vi "Fit Tilted Logistic Square Pulse.vi"(0 "Decay":T14, 5 "Boundaries":dbl[](array[numeric]), 9 "Basic Fit Options":T4, 11 "error in (no error)":errorcluster, 12 "Square Pulse Options":T2={"Method"=enum."Mode", "# Bins"=0, "Threshold %"=10.0, "Center on Midpoint"=TRUE, "Smoothen Plot"=FALSE}) -> (4 "Fitted Decay":cluster{"t Array":dbl[], "Fitted Array":dbl[]}, 6 "Residuals":cluster{"t Array":dbl[], "Residual Array":dbl[]}, 8 "Fit Output":T9={"best nonlinear fit"=[], "best fit parameters"=[], "R^2"=0.0, "RMSE"=0.0, "error out"={"status"=FALSE, "code"=0, "source"=""}, "Fitting Method"=enum."Least Square", "number of function calls"=0, "number of iterations"=0, "covariance"=[], "Chi 2"=0.0, "DOF"=0, "Fit Convergence Criterion"=enum."Continue", "Fitting Algorithm"=enum."Levenberg-Marquardt", "Weighted Fit"=enum."Unweighted", "Gradient"=0.0, "|Delta Chi 2|"=0.0, "|Delta Chi 2|/Chi 2"=0.0, "Max |Delta a| /|a|"=0.0, "Lambda"=-1.0, "RSS"=0.0, "AIC"=0.0, "BIC"=0.0, "Max number of function calls"=0, "Max number of iterations"=0, "IRF"={"X Array"=[], "Y Array"=[]}, "IRF Normalization Factor"=0.0, "Decay Normalization Factor"=0.0, "Number of offset fits"=0, "Weighted Chi2"=-1.0, "Unweighted Chi2"=-1.0}, 10 "Delta Best Fit Parameters":dbl[](array[numeric]), 15 "error out":errorcluster)   [LabVIEW 2021, in "Fits.lvlib"]
uses:
  Fits.lvlib
  Time/Time.lvlib
  <vilib>/ErrorRing/Error Ring.xnode
  <vilib>/Utility/error.llb/DialogType.ctl
  LM model Function and gradient (Tilted Logistic Square-Gated IRF).vi
  <vilib>/Utility/error.llb/Error Cluster From Error Code.vi
  Arrays/Arrays.lvlib
  Graphs/XY Graph/XY Graph Plot Data.ctl
  Graphs/XY Graph/XY Graph Add-Ons.lvlib
  Decay Convolution/Fit Control Data.ctl
  <vilib>/Analysis/Matrix/Datatypes/RealMatrix.ctl
  <vilib>/Analysis/Matrix/NI_Matrix.lvlib
  Non-linear Fit Output v4.ctl
  Residual Type.ctl
  Basic Fit Options.ctl
  Square Pulse Levels Type.ctl
  Square Pulse Options.ctl
  Convergence Criteria.ctl
  Non-linear Fitting Algorithm.ctl
  Non-linear Fitting Method v2.ctl
  Nonlinear Fit Method.ctl
  Optimal Offset Selection Criterion.ctl
  IRF(X)PSED/Fit Weights Type v2.ctl
panel:
  in  "Optimal Offset Selection Criterion":T1
  out "XY Graph":cluster{"X Array":dbl[], "Y Array":dbl[]}[](graph)
  out "CPU (s)":dbl
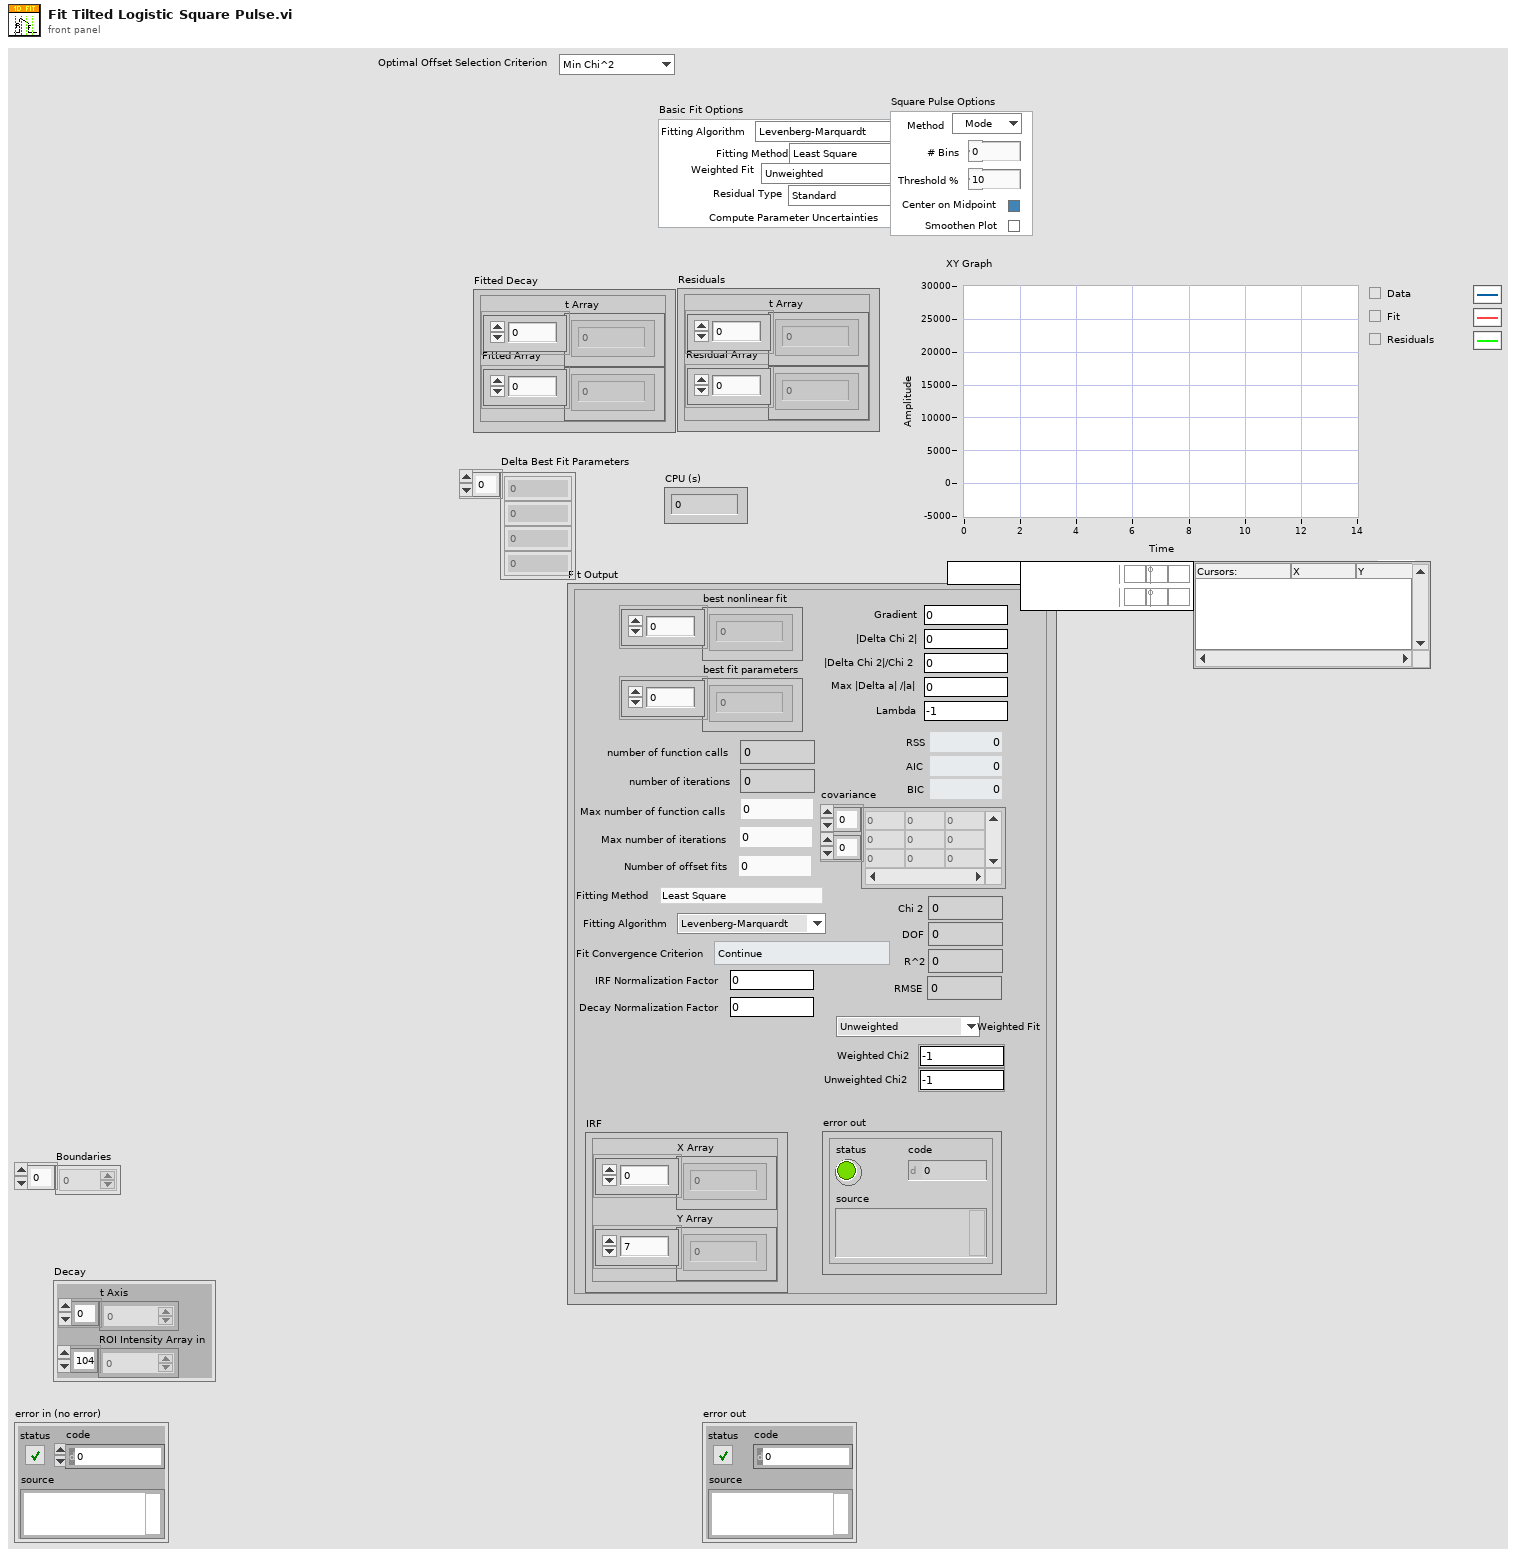
[diagram p1: front panel]
types:
  T1 = typedef "Fits.lvlib/Optimal Offset Selection Criterion.ctl" = enum16{"Min Chi^2", "Max R^2"}
  T2 = typedef "Fits.lvlib/Square Pulse Options.ctl" = cluster{"Method":T3, "# Bins":i32, "Threshold %":dbl, "Center on Midpoint":bool, "Smoothen Plot":bool}
  T3 = typedef "Fits.lvlib/Square Pulse Levels Type.ctl" = enum16{"Mode", "Mean"}
  T4 = typedef "Fits.lvlib/Basic Fit Options.ctl" = cluster{"Fitting Method":T5, "Weighted Fit":T6, "Residual Type":T7, "Compute Parameter Uncertainties":bool, "Fitting Algorithm":T8}
  T5 = typedef "Fits.lvlib/Non-linear Fitting Method v2.ctl" = enum16{"Least Square", "Least Absolute Residual", "Bisquare", "MLE", "-", "Best of All"}
  T6 = typedef "Fits.lvlib/Fit Weights Type v2.ctl" = enum16{"Unweighted", "1/Variance (Neyman)", "1/Variance (Pearson)", "Best of All"}
  T7 = typedef "Fits.lvlib/Residual Type.ctl" = enum16{"Standard", "Normalized", "Reduced"}
  T8 = typedef "Fits.lvlib/Non-linear Fitting Algorithm.ctl" = enum16{"Levenberg-Marquardt", "Trust-Region Dogleg"}
  T9 = typedef "Fits.lvlib/Non-linear Fit Output v4.ctl" = cluster{"best nonlinear fit":dbl[], "best fit parameters":dbl[], "R^2":dbl, "RMSE":dbl, "error out":errorcluster, "Fitting Method":T10, "number of function calls":i32, "number of iterations":i32, "covariance":T11, "Chi 2":dbl, "DOF":i32, "Fit Convergence Criterion":T12, "Fitting Algorithm":T8, "Weighted Fit":T6, "Gradient":dbl, "|Delta Chi 2|":dbl, "|Delta Chi 2|/Chi 2":dbl, "Max |Delta a| /|a|":dbl, "Lambda":dbl, "RSS":dbl, "AIC":dbl, "BIC":dbl, "Max number of function calls":i32, "Max number of iterations":i32, "IRF":T13, "IRF Normalization Factor":dbl, "Decay Normalization Factor":dbl, "Number of offset fits":i32, "Weighted Chi2":dbl, "Unweighted Chi2":dbl}
  T10 = typedef "Fits.lvlib/Nonlinear Fit Method.ctl" = enum16{"Least Square", "Least Absolute Residual", "Bisquare", "MLE"}
  T11 = typedef "NI_Matrix.lvlib/RealMatrix.ctl" = dbl[][]
  T12 = typedef "Fits.lvlib/Convergence Criteria.ctl" = enum16{"Continue", "Tolerances Exceeded", "Max Time Exceeded", "Max Iterations Exceeded", "Max Function Evaluations Exceeded", "Scale Range Exceeded"}
  T13 = typedef "XY Graph Add-Ons.lvlib/XY Graph Plot Data.ctl" = cluster{"X Array":dbl[], "Y Array":dbl[]}
  T14 = cluster{"t Axis":dbl[], "ROI Intensity Array in":dbl[]}
  T15 = cluster{"parameter minimum":dbl[], "parameter maximum":dbl[]}
  T16 = typedef "DialogType.ctl" = u16
  T17 = typedef "Fits.lvlib/Fit Control Data.ctl" = cluster{"IRF":T13, "Laser Period":dbl, "SYNC Period":dbl}
  T18 = cluster{"t Axis":dbl[], "best nonlinear fit":dbl[]}
  T19 = cluster{"t Axis":dbl[], "best nonlinear fit":dbl[]}[]
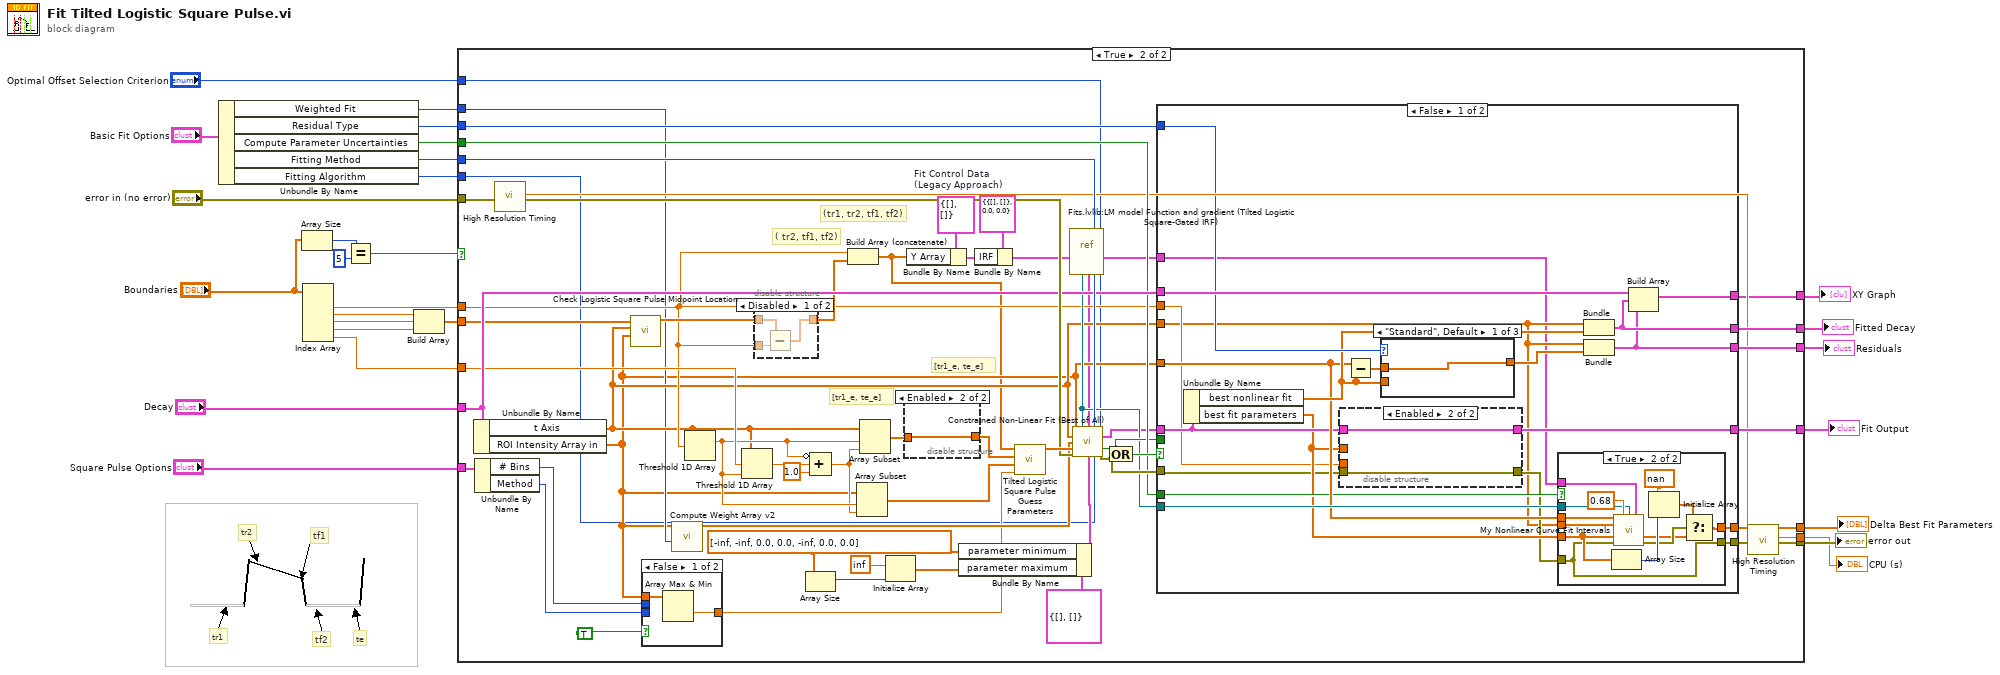
[diagram p0: block diagram]
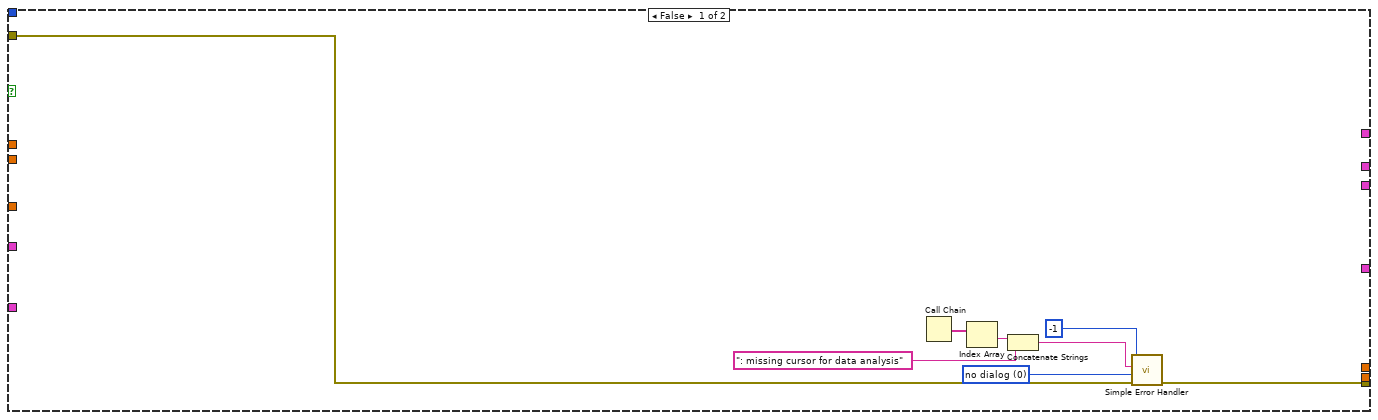
[diagram p2: hidden frame]
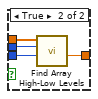
[diagram p3: hidden frame]
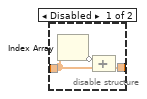
[diagram p5: hidden frame]
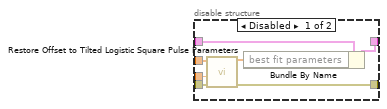
[diagram p6: hidden frame]
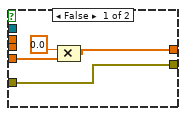
[diagram p7: hidden frame]
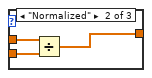
[diagram p8: hidden frame]
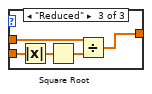
[diagram p9: hidden frame]
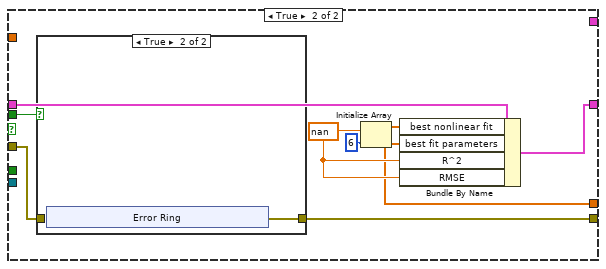
[diagram p10: hidden frame]
diagram:
  # "te"
  # "tf2"
  # "tf1"
  # "tr2"
  # "tr1"
  n1 = Unbundle By Name("Basic Fit Options") -> ("Weighted Fit"=w4:T6, "Residual Type"=w23:T7, "Compute Parameter Uncertainties"=w24:bool, "Fitting Method"=w26:T5, "Fitting Algorithm"=w2:T8)
  n2 = Array Size(array="Boundaries") -> (size(s)=w14:i32)
  n3 = Index Array(array="Boundaries") -> (element #1=w15:dbl, element #2=w12:dbl, element #3=w11:dbl, element #4=w10:dbl, element #5=w9:dbl)  [unwired: 5 in]
  n4 = Equal?(x=w14, y=5) -> (x = y?=w8:bool)
  n5 = Build Array(w12, w11, w10) -> (w27:dbl[])
  n6 = case shown="True" w8 {
    tunnel: w27 -> [_ w56]
    tunnel: "error in (no error)" -> [w29 w89]
    tunnel: w26 -> [_ w88]
    tunnel: "Decay" -> [_ w81]
    tunnel: w24 -> [_ w80]
    tunnel: w23 -> [_ w79]
    tunnel: [_ w76] -> w22
    tunnel: [_ w75] -> w21
    tunnel: [_ w74] -> w20
    tunnel: [_ w73] -> w19
    tunnel: [w35 w72] -> w18
    tunnel: [_ w71] -> w17
    tunnel: [_ w69] -> w16
    tunnel: w15 -> [_ w53]
    tunnel: w9 -> [_ w68]
    tunnel: w4 -> [_ w51]
    tunnel: "Square Pulse Options" -> [_ w49]
    tunnel: w2 -> [_ w43]
    tunnel: "Optimal Offset Selection Criterion" -> [_ w41]
    frame False {
      w34 = T16 0 items=["no dialog", "OK message", "continue or stop message", "OK message + warnings", "continue/stop + warnings"] ("type of dialog (OK msg:1)")
      n7 = Call Chain() -> (call chain=w33:string[])
      n8 = Index Array(array=w33) -> (element=w32:string)  [unwired: 1 in]
      n9 = Concatenate Strings(w32, ": missing cursor for data analysis" ("format string")) -> (w30:string)
      n10 = call <vilib>:"Simple Error Handler.vi"("error code (no error:0)"=-1, "error source (\" \")"=w30, "type of dialog (OK msg:1)"=w34, "error in (no error)"=w29) -> ("error out"=w35:errorcluster)  [unwired: 1 in, 4 out]
    }
    frame True {
      w40 = T17 {"IRF"={"X Array"=[], "Y Array"=[]}, "Laser Period"=0.0, "SYNC Period"=0.0}  # Fit Control Data (Legacy Approach)
      w61 = dbl[] [-inf, -inf, 0.0, 0.0, -inf, 0.0, 0.0] ("parameter minimum")
      # "(tr1, tr2, tf1, tf2)"
      # "[tr1_e, te_e]"
      # "( tr2, tf1, tf2)"
      # "[tr1_e, te_e]"
      n11 = Unbundle By Name(w81) -> ("t Axis"=w52:dbl[], "ROI Intensity Array in"=w45:dbl[])
      n12 = Unbundle By Name(w49) -> ("# Bins"=w47:i32, "Method"=w46:T3)
      n13 = call "High Resolution Timing.vi"("Error In"=w89) -> ("elapsed (relative) seconds"=w70:dbl, "Error Out"=w87:errorcluster)  [unwired: 16 in, 1 out]
      n14 = call "Check Logistic Square Pulse Midpoint Location.vi"("Amplitude Array"=w45, "t Array"=w52, "Cursors in"=w56) -> ("Cursors out"=w55:dbl[])  [unwired: 8 in]
      n15 = case shown="False" TRUE {
        tunnel: [w91 w96] -> w44
        tunnel: w46 -> [_ w95]
        tunnel: w47 -> [_ w94]
        tunnel: w45 -> [w92 w93]
        frame False {
          n16 = Array Max & Min(array=w92) -> (min value=w91:dbl)  [unwired: 3 out]
        }
        frame True {
          n17 = call "Find Array High-Low Levels.vi"("Method (Mode)"=w95, "# Bins (auto)"=w94, "Array"=w93) -> ("Low Level"=w96:dbl)  [unwired: 6 in, 2 out]
        }
      }
      n18 = call "Compute Weight Array v2.vi"("Weighted Fit"=w51, "Data Array"=w45) -> ("Weight Array"=w50:dbl[])  [unwired: 8 in, 1 out]
      n19 = Threshold 1D Array(2:w53, 3:w52) -> (0:w66:dbl)  [unwired: 1 in]
      n20 = Threshold 1D Array(1:w66, 2:w68, 3:w52) -> (0:w67:dbl)
      n21 = disable-structure shown="Disabled" {
        disable-tunnel: w53 -> [w99 _]
        disable-tunnel: [w98 w100] -> w57
        disable-tunnel: w55 -> [w97 w100]
        frame Disabled {
          n22 = Subtract(x=w97, y=w99) -> (x-y=w98:dbl[])
        }
        frame Enabled {
        }
      }
      n23 = Array Size(array=w61) -> (size(s)=w62:i32)
      n24 = Compound Arithmetic op=ADD(invert w66, w67, 1.0 ("value")) -> (w64:dbl)
      n25 = Build Array (concatenate)(w53, w57) -> (w37:dbl[])
      n26 = Array Subset(array=w45, index=w66, length=w64) -> (w59:dbl[])
      n27 = Array Subset(array=w52, index=w66, length=w64) -> (w84:dbl[])
      n28 = Initialize Array(inf ("Numeric"), w62) -> (w60:dbl[])
      n29 = disable-structure shown="Enabled" {
        disable-tunnel: w84 -> [w103 w104]
        disable-tunnel: [w101 w104] -> w58
        frame Disabled {
          n30 = Index Array(array=w103) -> (element=w102:dbl)  [unwired: 1 in]
          n31 = Compound Arithmetic op=ADD(invert w102, w103) -> (w101:dbl[])
        }
        frame Enabled {
        }
      }
      n32 = Bundle By Name(cluster=T13 {"X Array"=[], "Y Array"=[]} ("IRF"), "Y Array"=w37) -> (w38:T13)
      n33 = Bundle By Name(cluster=T15 {"parameter minimum"=[], "parameter maximum"=[]} ("parameter bounds"), "parameter minimum"=w61, "parameter maximum"=w60) -> (w86:T15)
      n34 = Bundle By Name(cluster=w40, "IRF"=w38) -> (w36:T17)
      n35 = call "Tilted Logistic Square Pulse Guess Parameters.vi"("A_L"=w44, "F Array"=w59, "t Array"=w58, "tr1, tr2, tf1, tf2"=w37) -> ("Guess Parameters"=w90:dbl[])  [unwired: 7 in]
      n36 = vi-ref "Fits.lvlib:LM model Function and gradient (Tilted Logistic Square-Gated IRF).vi"() -> (w54:refnum<vi>)
      n37 = call "Constrained Non-Linear Fit (Best of All).vi"("Y Array"=w45, "f(x,a)"=w54, "Data"=w36, "Fitting Method"=w88, "Optimal Offset Selection Criterion"=w41, "X Array"=w52, "Weights"=w50, "Guess Fitted Parameters"=w90, "error in (no error)"=w87, "Fitted parameter bounds"=w86, "Fitting Algorithm"=w43) -> ("Fit Output"=w42:T9, "Fit Aborted?"=w78:bool, "Error Out"=w82:errorcluster)  [unwired: 1 in, 1 out]
      n38 = Compound Arithmetic op=OR(w78, w82) -> (w83:bool)
      n39 = case shown="False" w83 {
        tunnel: w81 -> [w125 _]
        tunnel: [w124 _] -> w69
        tunnel: [w123 _] -> w74
        tunnel: [w122 w166] -> w77
        tunnel: [w121 w162] -> w73
        tunnel: [w120 _] -> w75
        tunnel: w79 -> [w119 _]
        tunnel: w52 -> [w106 _]
        tunnel: w54 -> [w116 _]
        tunnel: w45 -> [w114 _]
        tunnel: w42 -> [w113 w165]
        tunnel: w82 -> [w110 w167]
        tunnel: [w108 w164] -> w76
        tunnel: w80 -> [w112 _]
        tunnel: w78 -> [_ w161]
        tunnel: w53 -> [w107 _]
        tunnel: w36 -> [w105 _]
        frame False {
          n40 = Unbundle By Name(w113) -> ("best nonlinear fit"=w115:dbl[], "best fit parameters"=w111:dbl[])
          n41 = disable-structure shown="Enabled" {
            disable-tunnel: w113 -> [w132 w134]
            disable-tunnel: w111 -> [w131 _]
            disable-tunnel: w110 -> [w130 w133]
            disable-tunnel: [w129 w133] -> w109
            disable-tunnel: [w128 w134] -> w108
            disable-tunnel: w107 -> [w126 _]
            frame Disabled {
              n42 = call "Restore Offset to Tilted Logistic Square Pulse Parameters.vi"("Error In"=w130, "Offset"=w126, "Best Fit Parameters"=w131) -> ("Error Out"=w129:errorcluster, "Offset Best Fit Parameters"=w127:dbl[])  [unwired: 7 in]
              n43 = Bundle By Name(cluster=w132, "best fit parameters"=w127) -> (w128:T9)
            }
            frame Enabled {
            }
          }
          n44 = Subtract(x=w114, y=w115) -> (x-y=w118:dbl[])
          n45 = case shown="\"Standard\", Default" w119 {
            tunnel: w118 -> [w152 w155 w160]
            tunnel: [w152 w153 w158] -> w117
            tunnel: w115 -> [_ w154 w159]
            frame "Standard", Default {
            }
            frame "Normalized" {
              n46 = Divide(x=w155, y=w154) -> (x/y=w153:dbl[])
            }
            frame "Reduced" {
              n47 = Absolute Value(x=w159) -> (abs(x)=w157:dbl[])
              n48 = Square Root(x=w157) -> (sqrt(x)=w156:dbl[])
              n49 = Divide(x=w160, y=w156) -> (x/y=w158:dbl[])
            }
          }
          n50 = case shown="True" w112 {
            tunnel: [w138 w139] -> w122
            tunnel: [w136 w140] -> w121
            tunnel: w106 -> [_ w150]
            tunnel: w116 -> [_ w149]
            tunnel: w105 -> [_ w148]
            tunnel: w111 -> [w137 w146]
            tunnel: w114 -> [_ w147]
            tunnel: w109 -> [w138 w139]
            frame False {
              n51 = Compound Arithmetic op=MULTIPLY(0.0, w137) -> (w136:dbl[])
            }
            frame True {
              n52 = Array Size(array=w146) -> (size(s)=w145:i32)
              n53 = call "My Nonlinear Curve Fit Intervals.vi"("Y"=w147, "confidence level"=0.68, "f(x,a)"=w149, "data"=w148, "X"=w150, "best fit parameters"=w146, "error in (no error)"=w139) -> ("delta best fit parameters"=w141:dbl[], "error out"=w142:errorcluster)  [unwired: 7 in]
              n54 = Initialize Array(nan ("element"), w145) -> (w143:dbl[])
              n55 = Select(t=w143, s=w142, f=w141) -> (s? t:f=w140:dbl[])
            }
          }
          n56 = Bundle("t Axis"=w106, "best nonlinear fit"=w115) -> (w123:T18)  [unwired: 1 in]
          n57 = Bundle("t Axis"=w106, w117) -> (w120:cluster{"t Axis":dbl[], dbl[]})  [unwired: 1 in]
          n58 = Build Array(w125, w123, w120) -> (w124:T19)
        }
        frame True {
          w163 = nan ("element")
          n59 = case shown="True" w161 {
            tunnel: w167 -> [w169 _]
            tunnel: [w169 w170] -> w166
            frame False {
            }
            frame True {
              n60 = xnode "Error Ring"() -> ("error out"=w170:errorcluster)
            }
          }
          n61 = Initialize Array(w163, 6 ("dimension size")) -> (w162:dbl[])
          n62 = Bundle By Name(cluster=w165, "best nonlinear fit"=w162, "best fit parameters"=w162, "R^2"=w163, "RMSE"=w163) -> (w164:T9)
        }
      }
      n63 = call "High Resolution Timing.vi"("relative seconds (NaN)"=w70, "Error In"=w77) -> ("elapsed (relative) seconds"=w71:dbl, "Error Out"=w72:errorcluster)  [unwired: 15 in, 1 out]
    }
  }
  "error out" <- w18
  "Fit Output" <- w22
  "Residuals" <- w21
  "Fitted Decay" <- w20
  "Delta Best Fit Parameters" <- w19
  "CPU (s)" <- w17
  "XY Graph" <- w16
